vi "Auto Detect UI.vi"(8 "error in (no error)":errorcluster, 11 "RP2040.lvlib:RP2040Platform in":refnum<class "RP2040Platform.lvclass">) -> (0 "error out":errorcluster, 1 "Cancelled":bool, 2 "Resource":refnum<class "DeployResource.lvclass">, 3 "RP2040.lvlib:RP2040Platform out":refnum<class "RP2040Platform.lvclass">)   [LabVIEW 2020, in "RP2040.lvlib" / "RP2040Platform.lvclass"]
uses:
  RP2040Platform.lvclass
  Builds/picoG/ppl/PicoG-Core.lvlibp/DeployResource/DeployResource.lvclass
  VisaResource/VisaResource.lvclass
  C:/dev/Vireo/PicoG/Builds/picoG/ppl/PicoG-Core.lvlibp/DeployResource/DeployResource.lvclass
panel:
  in  "Resources":i32(listbox)
  in  "Cancel":bool
  in  "OK":bool
  # "Reset and select your Pi Pico"
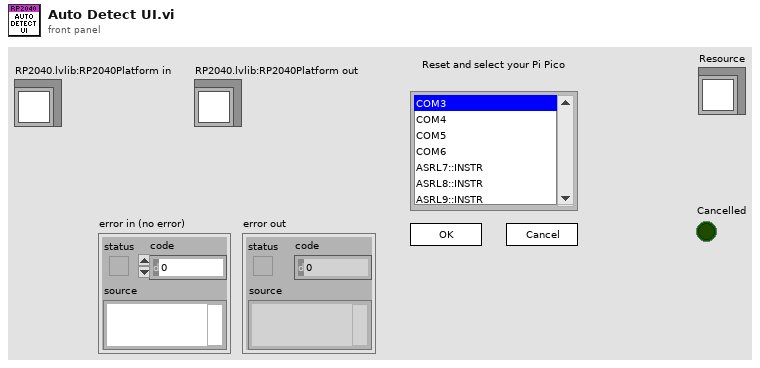
[diagram p1: front panel]
types:
  T1 = enum8{"Enabled", "Disabled", "Disabled and Grayed Out"}
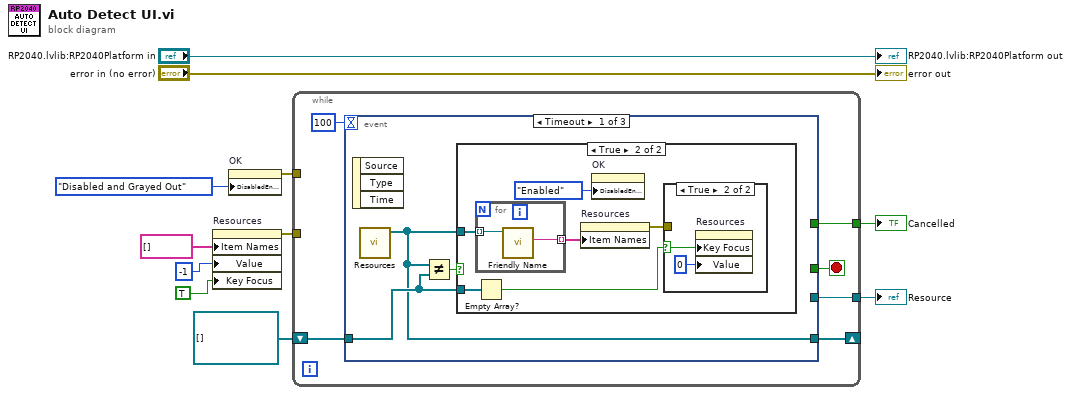
[diagram p0: block diagram]
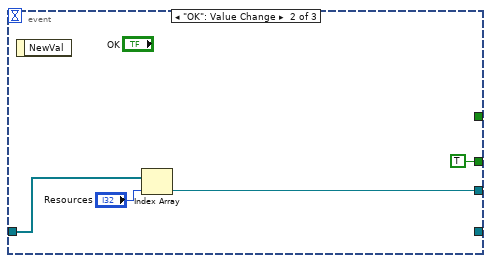
[diagram p4: hidden frame]
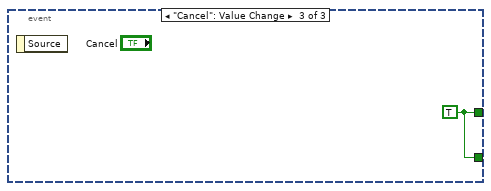
[diagram p5: hidden frame]
diagram:
  n1 = property on="Resources" class="LstBox (strict)"("Item Names"=string[] [], "Value"=-1 ("Resources"), "Key Focus"=TRUE) -> (error out=w2:errorcluster)  [unwired: 2 in, 1 out]
  n2 = property on="OK" class="Bool"("DisabledEnum"=T1."Disabled and Grayed Out" ("Disabled")) -> (error out=w8:errorcluster)  [unwired: 2 in, 1 out]
  n3 = while {
    shift-right: [w15] -> _
    shift-left: refnum<class "VisaResource.lvclass">[] [] ("Resources") -> [w16]
    tunnel: [w14] -> w10
    tunnel: w8 -> [_]
    tunnel: [w12] -> w3
    tunnel: w2 -> [_]
    stop <- w13 stop-if-true
    n4 = event shown="[0] Timeout" {
      selector: _ -> [_ _ _]
      dyn-events: _ -> [_ _ _]
      timeout: 100 -> [_ _ _]
      tunnel: w16 -> [w19 w32 _]
      tunnel: [w18 _ _] -> w15
      tunnel: [_ _ w35] -> w14
      tunnel: [_ TRUE w35] -> w13
      tunnel: [_ w31 _] -> w12
      event Timeout {
        n5 = event-data() -> ()  [unwired: 1 in, 3 out]
        n6 = call "Resources.vi"() -> ("Resources"=w18:refnum<class "VisaResource.lvclass">[])  [unwired: 11 in]
        n7 = Not Equal?(x=w18, y=w19) -> (x != y?=w20:bool)
        n8 = case shown="True" w20 {
          tunnel: w19 -> [_ w24]
          tunnel: w18 -> [_ w26]
          frame False {
          }
          frame True {
            n9 = for {
              tunnel: w26 -> [w30] mode=indexing
              tunnel: [w29] -> w25 mode=indexing
              n10 = call-dynamic "Friendly Name.vi"("VisaResource in"=w30) -> ("Friendly Name"=w29:string)  [unwired: 8 in, 2 out]
            }
            n11 = Empty Array?(array=w24) -> (empty?=w22:bool)
            n12 = property on="Resources" class="LstBox (strict)"("Item Names"=w25) -> (error out=w23:errorcluster)  [unwired: 2 in, 1 out]
            n13 = property on="OK" class="Bool"("DisabledEnum"=T1."Enabled" ("Disabled")) -> ()  [unwired: 2 in, 2 out]
            n14 = case shown="True" w22 {
              selector: w22 -> [_ w28]
              tunnel: w23 -> [_ _]
              frame False {
              }
              frame True {
                n15 = property on="Resources" class="LstBox (strict)"("Key Focus"=w28, "Value"=0 ("Resources")) -> ()  [unwired: 2 in, 2 out]
              }
            }
          }
        }
      }
      event "OK": Value Change {
        n16 = event-data() -> ()  [unwired: 1 in, 1 out]
        n17 = Index Array(array=w32, index="Resources") -> (element=w31:refnum<class "VisaResource.lvclass">)
      }
      event "Cancel": Value Change {
        w35 = TRUE
        n18 = event-data() -> ()  [unwired: 1 in, 1 out]
      }
    }
  }
  "Cancelled" <- w10
  "Resource" <- w3
  "error out" <- "error in (no error)"
  "RP2040.lvlib:RP2040Platform out" <- "RP2040.lvlib:RP2040Platform in"
